vi "configuration UI.vi"() -> ()   [LabVIEW 2014, in "Simple Sequencer TBM editor node.lvclass"]
doc: "This implements the main subpanel functionality for plugging into the Standard Configuration Editor."
uses:
  Simple Sequencer TBM editor node.lvclass
  <vilib>/NI/Configuration Framework/Node/NodeRef.ctl
  <vilib>/NI/Configuration Framework/Node/NISE_CEF_Node.lvclass
  <vilib>/NI/AMC/Message Queue.ctl
  <vilib>/NI/AMC/Message.ctl
  <vilib>/NI/Tools/Keyed Array/KeyedArray.ctl
  <vilib>/NI/Configuration Framework/Node/UserEventRef.ctl
  <vilib>/NI/Configuration Framework/Controls/EventCluster.ctl
  module/configuration/Simple Sequencer TBM configuration.lvclass
  user event typedef.ctl
  VI calling template typedef.ctl
  subpanel state.ctl
  action config and UI pairing.ctl
  sequencer parent classes/action configuration parent/action configuration.lvclass
  module/configuration/Simple Sequencer TBM configuration.lvclass/Simple Sequencer TBM configuration.ctl
  module/configuration/Read sequence definitions.vi
  module/configuration/Read sequencer name.vi
  module/configuration/Write sequencer name.vi
  module/configuration/Read supported actions list VI.vi
  <vilib>/NI/AMC/Create Single Message.vi
  <vilib>/NI/AMC/Update Message Routing Info.vi
  <vilib>/NI/Tag Bus Data Framework/Configuration Editor/Classes/Module editor node/Read Module Configuration.vi
  supported actions list template.vi
  <vilib>/NI/AMC/Send Message.vi
  <vilib>/NI/Tag Bus Module Framework/module configuration/TBM module configuration.lvclass
  <vilib>/NI/Configuration Framework/NISE_CEF_TreeControl.lvlib
  <vilib>/NI/AMC/AMC.lvlib
  <vilib>/NI/Tools/Keyed Array/Tools_KeyedArray.lvlib
panel:
  in  "Settings Button":bool
  in  "Shutdown Action":bool
  in  "Down Button":bool
  in  "Up Button":bool
  in  "Sequencer Name":string
  in  "delete action":bool
  in  "new action":bool
  in  "Actions":i32(listbox)
  in  "delete sequence":bool
  in  "new sequence":bool
  in  "Sequences":i32(listbox)
  in  "user event":T1
  in  "main queue":T2
  in  "node ref":T3
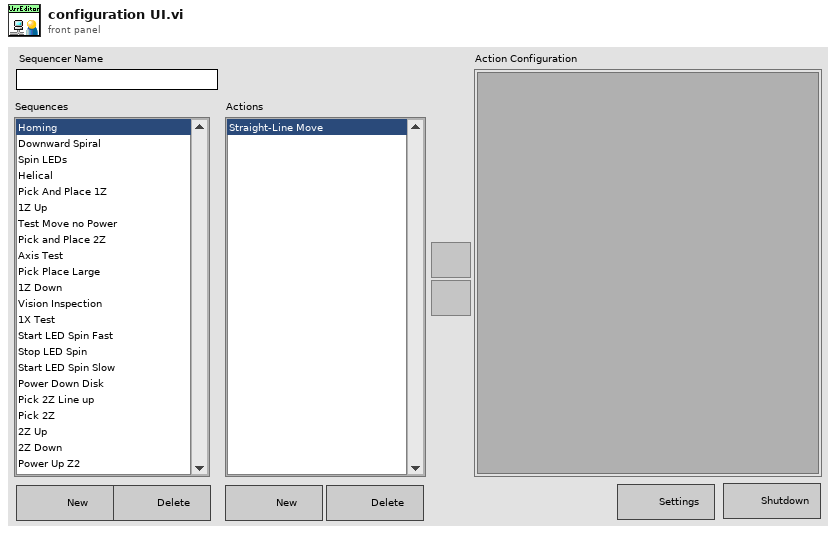
[diagram p1: front panel]
types:
  T1 = typedef "NISE_CEF_Node.lvclass/UserEventRef.ctl" = refnum<user-event>
  T2 = typedef "AMC.lvlib/Message Queue.ctl" = refnum<queue>
  T3 = typedef "NISE_CEF_Node.lvclass/NodeRef.ctl" = refnum<data-value>
  T4 = typedef "Simple Sequencer TBM editor node.lvclass/subpanel state.ctl" = cluster{"active VI":T5, "action UI user event":refnum<user-event>, "SubPnl Refnum":refnum<vi>, "supported actions list":T6[]}
  T5 = typedef "Simple Sequencer TBM editor node.lvclass/VI calling template typedef.ctl" = refnum<vi>
  T6 = typedef "Simple Sequencer TBM editor node.lvclass/action config and UI pairing.ctl" = cluster{"action config":refnum<class "action configuration.lvclass">, "display name":string, "UI VI Path":path}
  T7 = typedef "Simple Sequencer TBM editor node.lvclass/user event typedef.ctl" = cluster{"Message":string, "Data":string}
  T8 = typedef "NISE_CEF_TreeControl.lvlib/EventCluster.ctl" = cluster{"command":string, "data":string}
  T9 = enum8{"Enabled", "Disabled", "Disabled and Grayed Out"}
  T10 = typedef "Simple Sequencer TBM configuration.lvclass/sequence definition.ctl" = cluster{"sequence name":string, "action configs":refnum<class "action configuration.lvclass">[]}
  T11 = typedef "LVPoint32TypeDef.ctl" = cluster{"Horizontal":i32, "Vertical":i32}
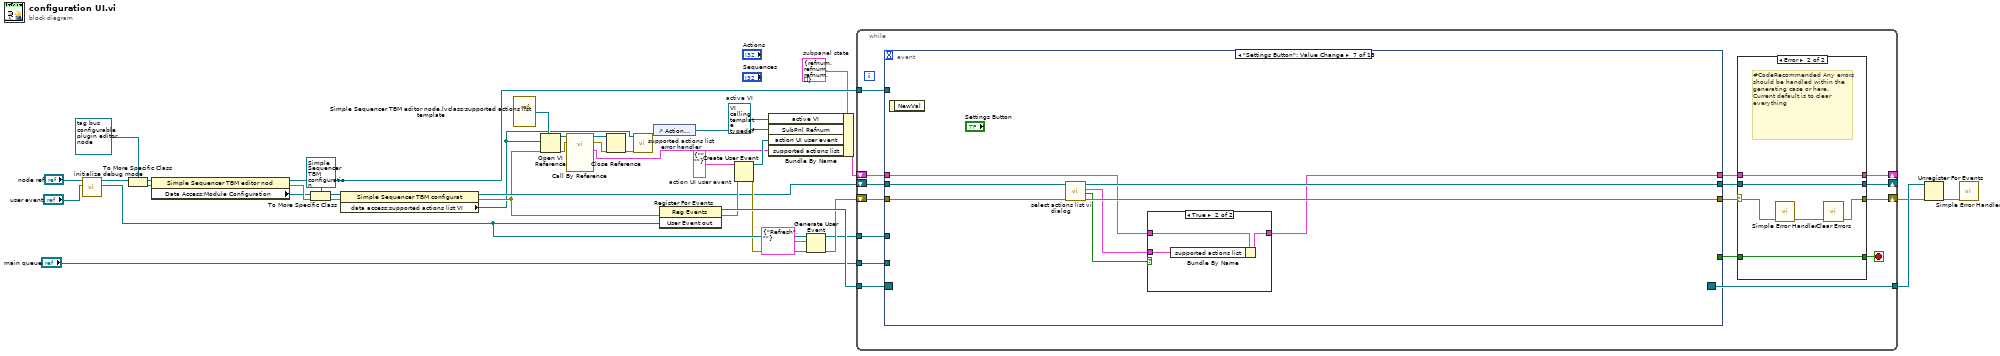
[diagram p0: block diagram]
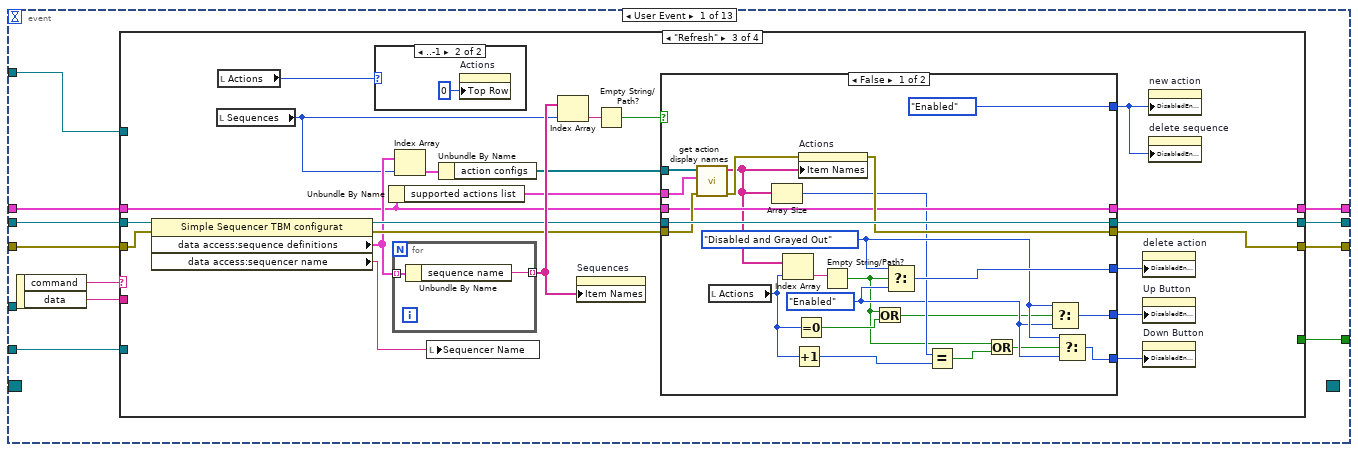
[diagram p3: hidden frame]
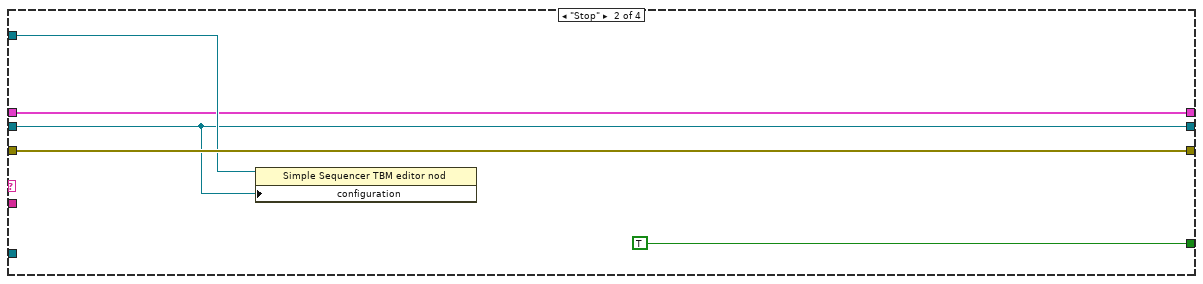
[diagram p5: hidden frame]
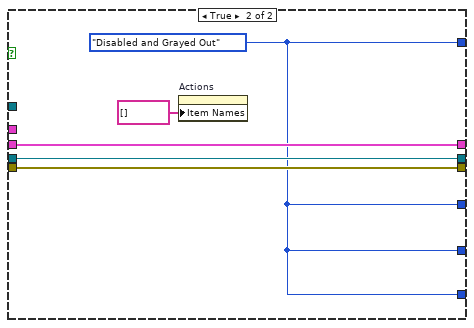
[diagram p7: hidden frame]
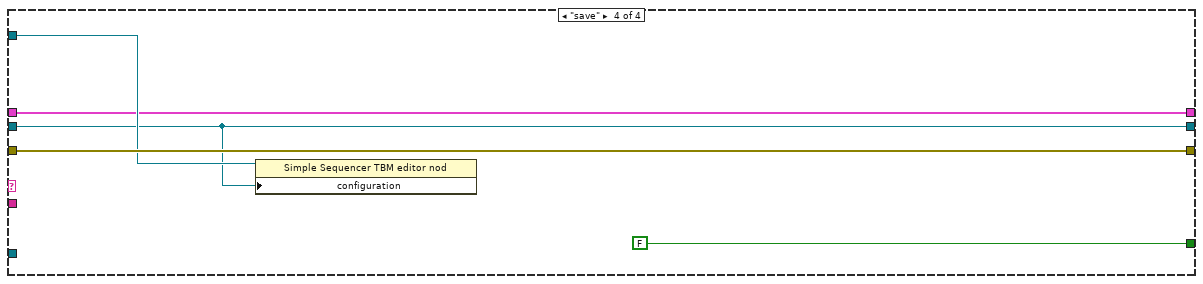
[diagram p8: hidden frame]
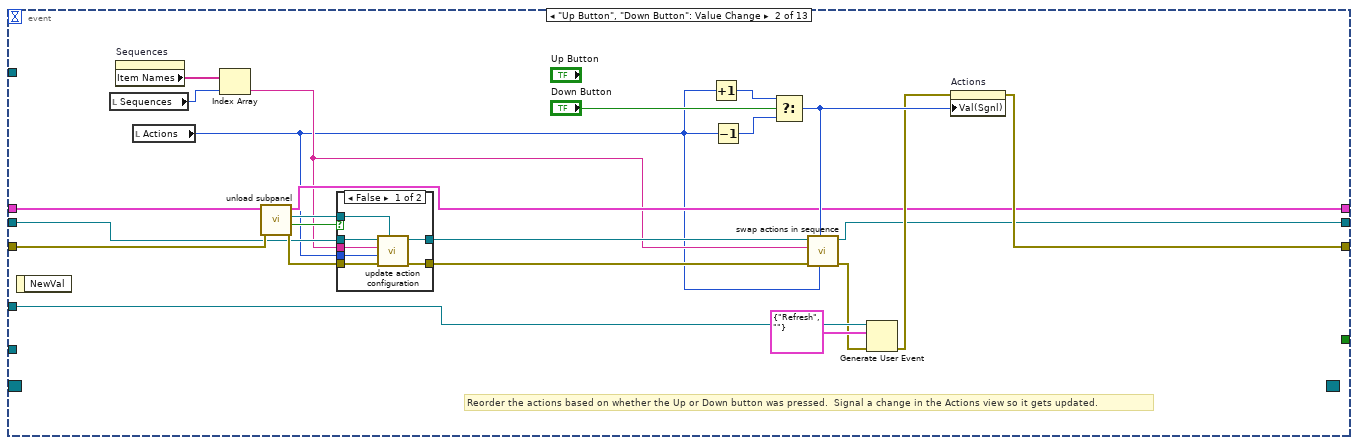
[diagram p9: hidden frame]
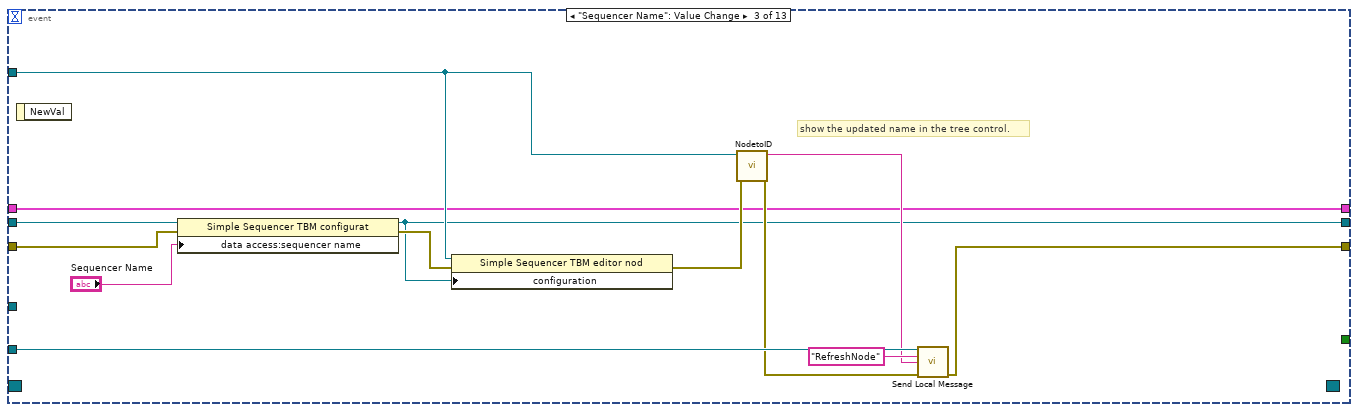
[diagram p11: hidden frame]
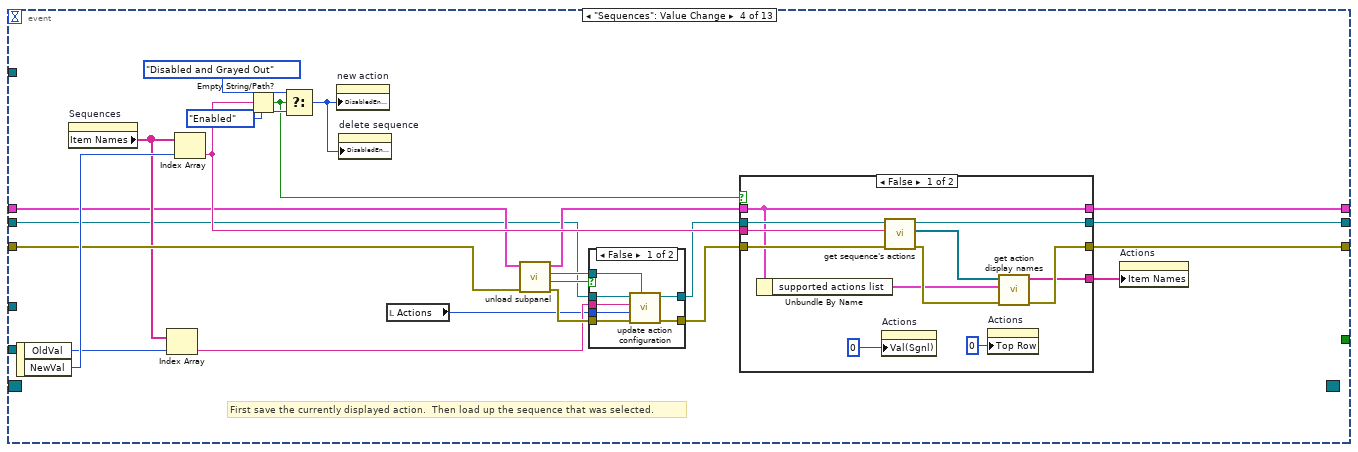
[diagram p12: hidden frame]
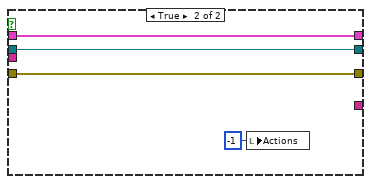
[diagram p14: hidden frame]
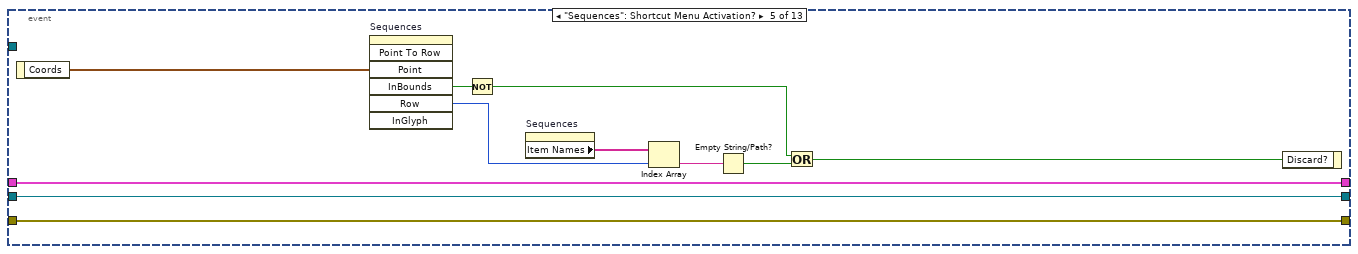
[diagram p15: hidden frame]
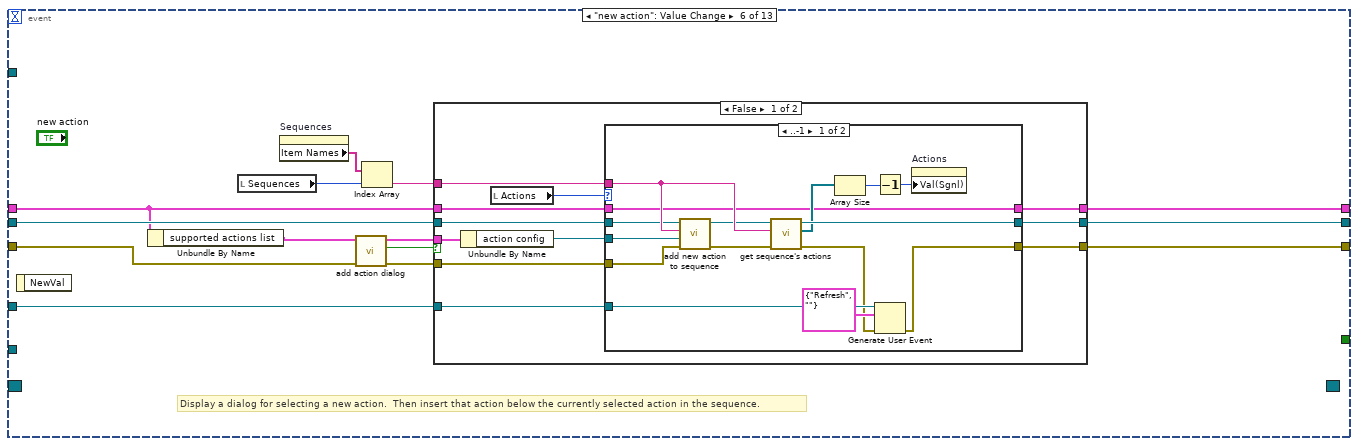
[diagram p16: hidden frame]
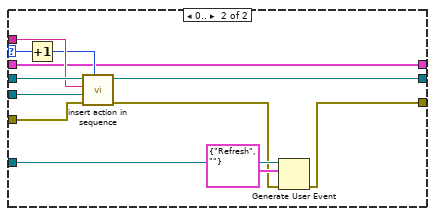
[diagram p17: hidden frame]
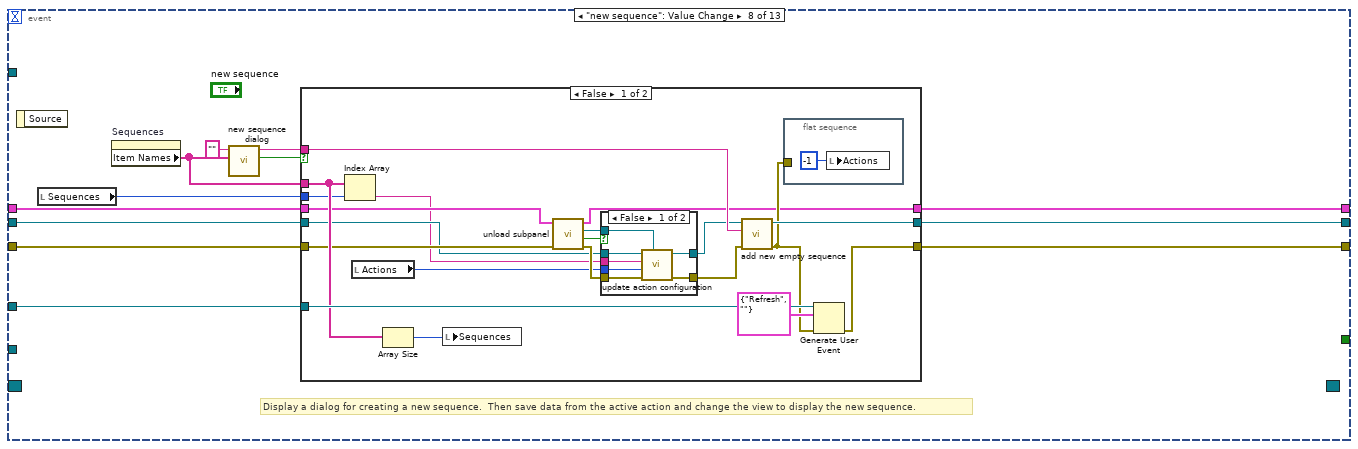
[diagram p20: hidden frame]
diagram:
  w16 = T4 {"active VI"=refnum, "action UI user event"=refnum, "SubPnl Refnum"=refnum, "supported actions list"=[]}  # subpanel state
  w22 = T5 refnum  # active VI
  w23 = T7 {"Message"="", "Data"=""}  # action UI user event
  n1 = call "initialize debug mode.vi"("User Event in"="user event", "editor node in"="node ref") -> ("User Event out"=w27:T1, "editor node out"=w18:T3)  [unwired: 7 in, 1 out]
  n2 = To More Specific Class(target class=refnum<data-value> refnum ("data value reference"), reference=w18) -> (specific class reference=w34:refnum<data-value>, error out=w33:errorcluster)  [unwired: 1 in]
  n3 = property class="Simple Sequencer TBM editor nod"(reference=w34, error in=w33) -> (reference out=w31:refnum<data-value>, error out=w17:errorcluster, "Data Access:Module Configuration"=w10:refnum<class "TBM module configuration.lvclass">)
  n4 = To More Specific Class(target class=refnum<class "Simple Sequencer TBM configuration.lvclass"> refnum ("user module configuration"), reference=w10, error in=w17) -> (specific class reference=w9:refnum<class "Simple Sequencer TBM configuration.lvclass">, error out=w8:errorcluster)
  n5 = property class="Simple Sequencer TBM configurat"(reference=w9, error in=w8) -> (reference out=w7:refnum<class "Simple Sequencer TBM configuration.lvclass">, error out=w6:errorcluster, "data access:supported actions list VI"=w1:path)
  n6 = vi-ref "Simple Sequencer TBM editor node.lvclass:supported actions list template.vi"() -> (w4:refnum<vi>)
  n7 = Open VI Reference(type specifier VI Refnum (for type only)=w4, vi path=w1, error in (no error)=w6) -> (vi reference=w12:refnum<vi>, error out=w3:errorcluster)  [unwired: 3 in]
  n8 = call-by-ref "?"(reference=w12, error in=w3) -> (reference out=w13:refnum<vi>, error out=w11:errorcluster, "supported actions list"=w5:T6[])  [unwired: 11 in]
  n9 = Close Reference(reference=w13, error in (no error)=w11) -> (error out=w2:errorcluster)
  n10 = call "supported actions list error handler.vi"("error in (no error)"=w2, "Path"=w1) -> ()  [unwired: 10 in]
  n11 = control-ref of="Action Configuration"() -> (w14:refnum<vi>)
  n12 = register-events(error in=w6, w27) -> (reference out=w39:refnum<event-registration>, error out=w21:errorcluster)  [unwired: 1 in]
  n13 = Create User Event(user event datatype=w23, error in=w21) -> (user event=w15:refnum<user-event>, error out=w20:errorcluster)
  n14 = Bundle By Name(cluster=w16, "active VI"=w22, "SubPnl Refnum"=w14, "action UI user event"=w15, "supported actions list"=w5) -> (w19:T4)
  n15 = Generate User Event(user event=w27, event data cluster=T8 {"command"="Refresh", "data"=""} ("event data"), error in=w20) -> (user event out=w24:T1, error out=w25:errorcluster)  [unwired: 1 in]
  n16 = while {
    tunnel: w39 -> [w55]
    tunnel: [w54] -> w38
    shift-right: [w50] -> w37
    shift-left: w25 -> [w53]
    shift-right: [w40] -> _
    shift-left: w7 -> [w49]
    tunnel: w31 -> [w47]
    tunnel: "main queue" -> [w46]
    tunnel: w24 -> [w45]
    shift-right: [w42] -> _
    shift-left: w19 -> [w44]
    stop <- w51 stop-if-true
    n17 = event shown="[6] \"Settings Button\": Value Change" {
      selector: w55 -> [_ _ _ _ _ _ _ _ _ _ _ _ _]
      dyn-events: [_ _ _ _ _ _ _ _ _ _ _ _ _] -> w54
      timeout: _ -> [_ _ _ _ _ _ _ _ _ _ _ _ _]
      tunnel: [w74 _ _ _ _ _ _ _ _ _ _ _ _] -> w41
      tunnel: [w75 w155 w184 w204 w246 w254 w306 w321 w363 w446 w499 w533 w572] -> w52
      tunnel: w53 -> [w76 w154 w182 w200 w246 w249 w308 w322 w365 w447 w494 w534 w583]
      tunnel: [w66 w143 w175 w205 w236 w251 w307 w314 w359 w441 w483 w510 w573] -> w48
      tunnel: w49 -> [w72 w149 w187 w192 w236 w250 w309 w323 w366 w448 w488 w517 w578]
      tunnel: w47 -> [w71 _ w177 _ _ _ _ _ _ _ _ _ _]
      tunnel: w46 -> [w70 _ w183 _ _ _ _ _ _ _ _ _ _]
      tunnel: w45 -> [_ w158 _ _ _ w253 _ w319 w362 w444 w498 _ w571]
      tunnel: w44 -> [w68 w153 w176 w197 w237 w248 w304 w318 w361 w443 w493 w521 w582]
      tunnel: [w67 w148 w176 w201 w237 w252 w302 w317 w360 w442 w489 w525 w570] -> w43
      event User Event {
        n18 = event-data() -> ("command"=w73:string, "data"=w69:string)  [unwired: 1 in]
        n19 = case shown="\"Refresh\"" w73 {
          tunnel: [_ TRUE _ FALSE] -> w74
          tunnel: w70 -> [_ _ _ _]
          tunnel: w72 -> [w78 w81 w105 w139]
          tunnel: w76 -> [w79 w83 w106 w141]
          tunnel: [w79 w83 w96 w141] -> w75
          tunnel: w71 -> [_ w82 _ w140]
          tunnel: w69 -> [_ _ _ _]
          tunnel: [w78 w81 w95 w139] -> w66
          tunnel: w68 -> [w77 w80 w86 w138]
          tunnel: [w77 w80 w92 w138] -> w67
          frame Default {
          }
          frame "Stop" {
            n20 = property class="Simple Sequencer TBM editor nod"(reference=w82, "configuration"=w81) -> ()  [unwired: 1 in, 2 out]
          }
          frame "Refresh" {
            n21 = property class="Simple Sequencer TBM configurat"(reference=w105, error in=w106) -> (reference out=w102:refnum<class "Simple Sequencer TBM configuration.lvclass">, error out=w101:errorcluster, "data access:sequence definitions"=w100:T10[], "data access:sequencer name"=w90:string)
            n22 = local read "Sequences"() -> (w99:i32)
            n23 = local read "Actions"() -> (w87:i32)
            n24 = case shown="..-1" w87 {
              frame 0.. {
              }
              frame ..-1 {
                n25 = property on="Actions" class="LstBox (strict)"("Top Row"=0) -> ()  [unwired: 2 in, 2 out]
              }
            }
            n26 = Unbundle By Name(w86) -> ("supported actions list"=w85:T6[])
            n27 = for {
              tunnel: w100 -> [w137] mode=indexing
              tunnel: [w136] -> w104 mode=indexing
              n28 = Unbundle By Name(w137) -> ("sequence name"=w136:string)
            }
            n29 = Index Array(array=w100, index=w99) -> (element=w98:T10)
            n30 = local write "Sequencer Name"(w90) -> ()
            n31 = Unbundle By Name(w98) -> ("action configs"=w97:refnum<class "action configuration.lvclass">[])
            n32 = Index Array(array=w104, index=w99) -> (element=w91:string)
            n33 = property on="Sequences" class="LstBox (strict)"("Item Names"=w104) -> ()  [unwired: 2 in, 2 out]
            n34 = Empty String/Path?(string/path=w91) -> (empty?=w103:bool)
            n35 = case shown="False" w103 {
              tunnel: [T9."Enabled" ("Disabled") w131] -> w94
              tunnel: w102 -> [w129 w135]
              tunnel: w101 -> [w126 w134]
              tunnel: w97 -> [w127 _]
              tunnel: [w125 w134] -> w96
              tunnel: [w129 w135] -> w95
              tunnel: [w123 w131] -> w93
              tunnel: w86 -> [w122 w132]
              tunnel: [w122 w132] -> w92
              tunnel: [w120 w131] -> w89
              tunnel: [w115 w131] -> w88
              tunnel: w85 -> [w108 _]
              frame False {
                w119 = T9."Disabled and Grayed Out" ("t")
                w114 = T9."Enabled" ("Disabled")
                n36 = call "get action display names.vi"("error in (no error)"=w126, "supported actions list"=w108, "action configs"=w127) -> ("error out"=w128:errorcluster, "display names"=w117:string[])  [unwired: 7 in]
                n37 = local read "Actions"() -> (w121:i32)
                n38 = Array Size(array=w117) -> (size(s)=w116:i32)
                n39 = Index Array(array=w117, index=w121) -> (element=w124:string)
                n40 = Increment(x=w121) -> (x+1=w118:i32)
                n41 = Equal To 0?(x=w121) -> (x = 0?=w113:bool)
                n42 = property on="Actions" class="LstBox (strict)"(error in=w128, "Item Names"=w117) -> (error out=w125:errorcluster)  [unwired: 1 in, 1 out]
                n43 = Empty String/Path?(string/path=w124) -> (empty?=w110:bool)
                n44 = Or(x=w110, y=w113) -> (x .or. y?=w112:bool)
                n45 = Select(t=w119, s=w110, f=w114) -> (s? t:f=w123:T9)
                n46 = Equal?(x=w116, y=w118) -> (x = y?=w111:bool)
                n47 = Or(x=w110, y=w111) -> (x .or. y?=w109:bool)
                n48 = Select(t=w119, s=w112, f=w114) -> (s? t:f=w120:T9)
                n49 = Select(t=w119, s=w109, f=w114) -> (s? t:f=w115:T9)
              }
              frame True {
                w131 = T9."Disabled and Grayed Out" ("Disabled")
                n50 = property on="Actions" class="LstBox (strict)"("Item Names"=string[] []) -> ()  [unwired: 2 in, 2 out]
              }
            }
            n51 = property on="delete action" class="Bool"("DisabledEnum"=w93) -> ()  [unwired: 2 in, 2 out]
            n52 = property on="Up Button" class="Bool"("DisabledEnum"=w89) -> ()  [unwired: 2 in, 2 out]
            n53 = property on="Down Button" class="Bool"("DisabledEnum"=w88) -> ()  [unwired: 2 in, 2 out]
            n54 = property on="new action" class="Bool"("DisabledEnum"=w94) -> ()  [unwired: 2 in, 2 out]
            n55 = property on="delete sequence" class="Bool"("DisabledEnum"=w94) -> ()  [unwired: 2 in, 2 out]
          }
          frame "save" {
            n56 = property class="Simple Sequencer TBM editor nod"(reference=w140, "configuration"=w139) -> ()  [unwired: 1 in, 2 out]
          }
        }
      }
      event "Up Button", "Down Button": Value Change {
        # "Reorder the actions based on whether the Up or Down button was pressed.  Signal a change in the Actions view so it gets updated."
        n57 = event-data() -> ()  [unwired: 1 in, 1 out]
        n58 = local read "Sequences"() -> (w161:i32)
        n59 = property on="Sequences" class="LstBox (strict)"() -> ("Item Names"=w162:string[])  [unwired: 2 in, 2 out]
        n60 = local read "Actions"() -> (w144:i32)
        n61 = Index Array(array=w162, index=w161) -> (element=w146:string)
        n62 = call "unload subpanel.vi"("error in (no error)"=w154, "subpanel state"=w153) -> ("error out"=w150:errorcluster, "empty?"=w151:bool, "action configuration out"=w152:refnum<class "action configuration.lvclass">, "subpanel state out"=w148:T4)  [unwired: 6 in]
        n63 = case shown="False" w151 {
          tunnel: w152 -> [w172 _]
          tunnel: w149 -> [w171 w174]
          tunnel: w144 -> [w170 _]
          tunnel: w146 -> [w169 _]
          tunnel: w150 -> [w168 w173]
          tunnel: [w167 w174] -> w147
          tunnel: [w166 w173] -> w145
          frame False {
            n64 = call "update action configuration.vi"("action config"=w172, "error in (no error)"=w168, "index"=w170, "sequence name"=w169, "Simple Sequencer TBM configuration in"=w171) -> ("error out"=w166:errorcluster, "Simple Sequencer TBM configuration out"=w167:refnum<class "Simple Sequencer TBM configuration.lvclass">)  [unwired: 5 in]
          }
          frame True {
          }
        }
        n65 = Increment(x=w144) -> (x+1=w165:i32)
        n66 = Decrement(x=w144) -> (x-1=w164:i32)
        n67 = Select(t=w165, s="Down Button", f=w164) -> (s? t:f=w160:i32)
        n68 = call "swap actions in sequence.vi"("action index 2"=w144, "action index 1"=w160, "error in (no error)"=w145, "sequence name"=w146, "Simple Sequencer TBM configuration in"=w147) -> ("error out"=w157:errorcluster, "Simple Sequencer TBM configuration out"=w143:refnum<class "Simple Sequencer TBM configuration.lvclass">)  [unwired: 5 in]
        n69 = Generate User Event(user event=w158, event data cluster=T8 {"command"="Refresh", "data"=""} ("event data"), error in=w157) -> (error out=w156:errorcluster)  [unwired: 1 in, 1 out]
        n70 = property on="Actions" class="LstBox (strict)"(error in=w156, "Val(Sgnl)"=w160) -> (error out=w155:errorcluster)  [unwired: 1 in, 1 out]
      }
      event "Sequencer Name": Value Change {
        # "show the updated name in the tree control."
        n71 = event-data() -> ()  [unwired: 1 in, 1 out]
        n72 = property class="Simple Sequencer TBM configurat"(reference=w187, error in=w182, "data access:sequencer name"="Sequencer Name") -> (reference out=w175:refnum<class "Simple Sequencer TBM configuration.lvclass">, error out=w179:errorcluster)
        n73 = property class="Simple Sequencer TBM editor nod"(reference=w177, error in=w179, "configuration"=w175) -> (error out=w178:errorcluster)  [unwired: 1 out]
        n74 = call <vilib>:"NodetoID.vi"("error in"=w178, "node ref"=w177) -> ("error out"=w181:errorcluster, "ID"=w180:string)  [unwired: 8 in]
        n75 = call <vilib>:"Send Local Message.vi"("message queue in"=w183, "message name"="RefreshNode", "message value"=w180, "error in"=w181) -> ("error out"=w184:errorcluster)  [unwired: 9 in, 2 out]
      }
      event "Sequences": Value Change {
        # "First save the currently displayed action.  Then load up the sequence that was selected."
        n76 = event-data() -> ("OldVal"=w198:i32, "NewVal"=w210:i32)  [unwired: 1 in]
        n77 = property on="Sequences" class="LstBox (strict)"() -> ("Item Names"=w199:string[])  [unwired: 2 in, 2 out]
        n78 = Index Array(array=w199, index=w198) -> (element=w189:string)
        n79 = Index Array(array=w199, index=w210) -> (element=w206:string)
        n80 = Empty String/Path?(string/path=w206) -> (empty?=w207:bool)
        n81 = Select(t=T9."Disabled and Grayed Out" ("Disabled"), s=w207, f=T9."Enabled" ("Disabled")) -> (s? t:f=w203:T9)
        n82 = property on="new action" class="Bool"("DisabledEnum"=w203) -> ()  [unwired: 2 in, 2 out]
        n83 = property on="delete sequence" class="Bool"("DisabledEnum"=w203) -> ()  [unwired: 2 in, 2 out]
        n84 = local read "Actions"() -> (w188:i32)
        n85 = call "unload subpanel.vi"("error in (no error)"=w200, "subpanel state"=w197) -> ("error out"=w193:errorcluster, "empty?"=w195:bool, "action configuration out"=w194:refnum<class "action configuration.lvclass">, "subpanel state out"=w196:T4)  [unwired: 6 in]
        n86 = case shown="False" w195 {
          tunnel: w194 -> [w217 _]
          tunnel: w192 -> [w216 w219]
          tunnel: w188 -> [w215 _]
          tunnel: w189 -> [w214 _]
          tunnel: w193 -> [w213 w218]
          tunnel: [w212 w219] -> w191
          tunnel: [w211 w218] -> w190
          frame False {
            n87 = call "update action configuration.vi"("action config"=w217, "error in (no error)"=w213, "index"=w215, "sequence name"=w214, "Simple Sequencer TBM configuration in"=w216) -> ("error out"=w211:errorcluster, "Simple Sequencer TBM configuration out"=w212:refnum<class "Simple Sequencer TBM configuration.lvclass">)  [unwired: 5 in]
          }
          frame True {
          }
        }
        n88 = case shown="False" w207 {
          tunnel: w191 -> [w223 w235]
          tunnel: w206 -> [w231 _]
          tunnel: w190 -> [w230 w234]
          tunnel: [w222 w235] -> w205
          tunnel: [w227 w234] -> w204
          tunnel: [w226 _] -> w202
          tunnel: w196 -> [w221 w233]
          tunnel: [w221 w233] -> w201
          frame False {
            n89 = Unbundle By Name(w221) -> ("supported actions list"=w220:T6[])
            n90 = property on="Actions" class="LstBox (strict)"("Val(Sgnl)"=0 ("Actions")) -> ()  [unwired: 2 in, 2 out]
            n91 = call "get sequence's actions.vi"("error in (no error)"=w230, "sequence name"=w231, "Simple Sequencer TBM configuration in"=w223) -> ("error out"=w228:errorcluster, "action configs"=w229:refnum<class "action configuration.lvclass">[], "Simple Sequencer TBM configuration out"=w222:refnum<class "Simple Sequencer TBM configuration.lvclass">)  [unwired: 6 in]
            n92 = property on="Actions" class="LstBox (strict)"("Top Row"=0) -> ()  [unwired: 2 in, 2 out]
            n93 = call "get action display names.vi"("error in (no error)"=w228, "supported actions list"=w220, "action configs"=w229) -> ("error out"=w227:errorcluster, "display names"=w226:string[])  [unwired: 7 in]
          }
          frame True {
            n94 = local write "Actions"(-1 ("Actions")) -> ()
          }
        }
        n95 = property on="Actions" class="LstBox (strict)"("Item Names"=w202) -> ()  [unwired: 2 in, 2 out]
      }
      event "Sequences": Shortcut Menu Activation? {
        n96 = event-data() -> ("Coords"=w243:T11)  [unwired: 1 in]
        n97 = invoke on="Sequences" class="LstBox (strict)" method="Point To Row"("Point"=w243) -> ("InBounds"=w241:bool, "Row"=w242:i32)  [unwired: 6 in, 5 out]
        n98 = Not(x=w241) -> (.not. x?=w239:bool)
        n99 = property on="Sequences" class="LstBox (strict)"() -> ("Item Names"=w245:string[])  [unwired: 2 in, 2 out]
        n100 = Index Array(array=w245, index=w242) -> (element=w244:string)
        n101 = Empty String/Path?(string/path=w244) -> (empty?=w240:bool)
        n102 = Or(x=w239, y=w240) -> (x .or. y?=w238:bool)
        n103 = event-data("Discard?"=w238) -> ()  [unwired: 1 in, 1 out]
      }
      event "new action": Value Change {
        # "Display a dialog for selecting a new action.  Then insert that action below the currently selected action in the sequence."
        n104 = event-data() -> ()  [unwired: 1 in, 1 out]
        n105 = Unbundle By Name(w248) -> ("supported actions list"=w247:T6[])
        n106 = local read "Sequences"() -> (w256:i32)
        n107 = property on="Sequences" class="LstBox (strict)"() -> ("Item Names"=w257:string[])  [unwired: 2 in, 2 out]
        n108 = call "add action dialog.vi"("error in (no error)"=w249, "supported actions list"=w247) -> ("error out"=w260:errorcluster, "cancelled"=w259:bool, "config and UI pairing"=w258:T6)  [unwired: 7 in]
        n109 = Index Array(array=w257, index=w256) -> (element=w255:string)
        n110 = case shown="False" w259 {
          tunnel: w260 -> [w266 w300]
          tunnel: [w268 w301] -> w251
          tunnel: w250 -> [w267 w301]
          tunnel: w258 -> [w271 _]
          tunnel: w255 -> [w263 _]
          tunnel: [w269 w300] -> w254
          tunnel: w253 -> [w270 _]
          tunnel: w248 -> [w262 w299]
          tunnel: [w261 w299] -> w252
          frame False {
            n111 = Unbundle By Name(w271) -> ("action config"=w265:refnum<class "action configuration.lvclass">)
            n112 = local read "Actions"() -> (w264:i32)
            n113 = case shown="..-1" w264 {
              selector: w264 -> [_ w292]
              tunnel: w270 -> [w285 w297]
              tunnel: [w284 w296] -> w269
              tunnel: [w282 w289] -> w268
              tunnel: w267 -> [w274 w295]
              tunnel: w266 -> [w277 w294]
              tunnel: w265 -> [w276 w293]
              tunnel: w263 -> [w275 w291]
              tunnel: w262 -> [w272 w287]
              tunnel: [w272 w287] -> w261
              frame ..-1 {
                n114 = call "add new action to sequence.vi"("error in (no error)"=w277, "new action"=w276, "sequence name"=w275, "Simple Sequencer TBM configuration in"=w274) -> ("error out"=w278:errorcluster, "Simple Sequencer TBM configuration out"=w273:refnum<class "Simple Sequencer TBM configuration.lvclass">)  [unwired: 6 in]
                n115 = call "get sequence's actions.vi"("error in (no error)"=w278, "sequence name"=w275, "Simple Sequencer TBM configuration in"=w273) -> ("error out"=w283:errorcluster, "action configs"=w280:refnum<class "action configuration.lvclass">[], "Simple Sequencer TBM configuration out"=w282:refnum<class "Simple Sequencer TBM configuration.lvclass">)  [unwired: 6 in]
                n116 = Array Size(array=w280) -> (size(s)=w281:i32)
                n117 = Decrement(x=w281) -> (x-1=w279:i32)
                n118 = Generate User Event(user event=w285, event data cluster=T8 {"command"="Refresh", "data"=""} ("event data"), error in=w283) -> (error out=w284:errorcluster)  [unwired: 1 in, 1 out]
                n119 = property on="Actions" class="LstBox (strict)"("Val(Sgnl)"=w279) -> ()  [unwired: 2 in, 2 out]
              }
              frame 0.. {
                n120 = Increment(x=w292) -> (x+1=w290:i32)
                n121 = call "insert action in sequence.vi"("index"=w290, "error in (no error)"=w294, "new action"=w293, "sequence name"=w291, "Simple Sequencer TBM configuration in"=w295) -> ("error out"=w288:errorcluster, "Simple Sequencer TBM configuration out"=w289:refnum<class "Simple Sequencer TBM configuration.lvclass">)  [unwired: 5 in]
                n122 = Generate User Event(user event=w297, event data cluster=T8 {"command"="Refresh", "data"=""} ("event data"), error in=w288) -> (error out=w296:errorcluster)  [unwired: 1 in, 1 out]
              }
            }
          }
          frame True {
          }
        }
      }
      event "Settings Button": Value Change {
        n123 = event-data() -> ()  [unwired: 1 in, 1 out]
        n124 = call "select actions list vi dialog.vi"("error in (no error)"=w308, "sequencer configuration"=w309) -> ("error out"=w306:errorcluster, "success?"=w305:bool, "supported actions list"=w303:T6[], "sequencer configuration out"=w307:refnum<class "Simple Sequencer TBM configuration.lvclass">)  [unwired: 6 in]
        n125 = case shown="True" w305 {
          tunnel: w304 -> [w310 w313]
          tunnel: w303 -> [_ w312]
          tunnel: [w310 w311] -> w302
          frame False {
          }
          frame True {
            n126 = Bundle By Name(cluster=w313, "supported actions list"=w312) -> (w311:T4)
          }
        }
      }
      event "new sequence": Value Change {
        # "Display a dialog for creating a new sequence.  Then save data from the active action and change the view to display the new sequence."
        n127 = event-data() -> ()  [unwired: 1 in, 1 out]
        n128 = local read "Sequences"() -> (w315:i32)
        n129 = property on="Sequences" class="LstBox (strict)"() -> ("Item Names"=w316:string[])  [unwired: 2 in, 2 out]
        n130 = call "new sequence dialog.vi"("Existing Sequences"=w316, "Sequence Name"="") -> ("Canceled?"=w324:bool, "Sequence Name Out"=w320:string)  [unwired: 8 in]
        n131 = case shown="False" w324 {
          tunnel: w323 -> [w330 w358]
          tunnel: w322 -> [w338 w357]
          tunnel: [w341 w358] -> w314
          tunnel: [w344 w357] -> w321
          tunnel: w320 -> [w342 _]
          tunnel: w319 -> [w343 _]
          tunnel: w318 -> [w335 w356]
          tunnel: [w334 w356] -> w317
          tunnel: w316 -> [w340 _]
          tunnel: w315 -> [w339 _]
          frame False {
            n132 = Index Array(array=w340, index=w339) -> (element=w329:string)
            n133 = local read "Actions"() -> (w328:i32)
            n134 = Array Size(array=w340) -> (size(s)=w337:i32)
            n135 = local write "Sequences"(w337) -> ()
            n136 = call "unload subpanel.vi"("error in (no error)"=w338, "subpanel state"=w335) -> ("error out"=w331:errorcluster, "empty?"=w332:bool, "action configuration out"=w333:refnum<class "action configuration.lvclass">, "subpanel state out"=w334:T4)  [unwired: 6 in]
            n137 = case shown="False" w332 {
              tunnel: w333 -> [w352 _]
              tunnel: w330 -> [w351 w354]
              tunnel: w328 -> [w350 _]
              tunnel: w329 -> [w349 _]
              tunnel: w331 -> [w348 w353]
              tunnel: [w347 w354] -> w327
              tunnel: [w346 w353] -> w326
              frame False {
                n138 = call "update action configuration.vi"("action config"=w352, "error in (no error)"=w348, "index"=w350, "sequence name"=w349, "Simple Sequencer TBM configuration in"=w351) -> ("error out"=w346:errorcluster, "Simple Sequencer TBM configuration out"=w347:refnum<class "Simple Sequencer TBM configuration.lvclass">)  [unwired: 5 in]
              }
              frame True {
              }
            }
            n139 = call "add new empty sequence.vi"("error in (no error)"=w326, "sequence name"=w342, "Simple Sequencer TBM configuration in"=w327) -> ("error out"=w336:errorcluster, "Simple Sequencer TBM configuration out"=w341:refnum<class "Simple Sequencer TBM configuration.lvclass">)  [unwired: 7 in]
            n140 = flat-sequence {
              tunnel: w336 -> [_]
              frame #0 {
                n141 = local write "Actions"(-1 ("Actions")) -> ()
              }
            }
            n142 = Generate User Event(user event=w343, event data cluster=T8 {"command"="Refresh", "data"=""} ("event data"), error in=w336) -> (error out=w344:errorcluster)  [unwired: 1 in, 1 out]
          }
          frame True {
          }
        }
      }
      event "Sequences": Shortcut Menu Selection (User) {
        n143 = event-data() -> ("ItemTag"=w367:string, "Coords"=w364:T11)  [unwired: 1 in]
        n144 = case shown="Default" w367 {
          tunnel: w366 -> [w370 w379 w403]
          tunnel: w365 -> [w369 w378 w424]
          tunnel: w364 -> [_ w383 w425]
          tunnel: [w370 w376 w416] -> w359
          tunnel: [w369 w375 w414] -> w363
          tunnel: w362 -> [_ w374 _]
          tunnel: w361 -> [w368 w372 w407]
          tunnel: [w368 w371 w398] -> w360
          frame Default {
          }
          frame "Edit".. {
            n145 = invoke on="Sequences" class="LstBox (strict)" method="Point To Row"("Point"=w383) -> ("Row"=w384:i32)  [unwired: 6 in, 6 out]
            n146 = property on="Sequences" class="LstBox (strict)"(error in=w378) -> (error out=w377:errorcluster, "Item Names"=w382:string[])  [unwired: 1 in, 1 out]
            n147 = Index Array(array=w382, index=w384) -> (element=w373:string)
            n148 = call "new sequence dialog.vi"("Existing Sequences"=w382, "Sequence Name"=w373) -> ("Canceled?"=w381:bool, "Sequence Name Out"=w380:string)  [unwired: 8 in]
            n149 = case shown="False" w381 {
              tunnel: w380 -> [w386 _]
              tunnel: w379 -> [w391 w397]
              tunnel: w377 -> [w389 w396]
              tunnel: [w390 w397] -> w376
              tunnel: [w393 w396] -> w375
              tunnel: w374 -> [w392 _]
              tunnel: w373 -> [w387 _]
              tunnel: w372 -> [w385 w395]
              tunnel: [w385 w395] -> w371
              frame False {
                n150 = call "rename sequence.vi"("error in (no error)"=w389, "new sequence name"=w386, "old sequence name"=w387, "Simple Sequencer TBM configuration in"=w391) -> ("error out"=w388:errorcluster, "Simple Sequencer TBM configuration out"=w390:refnum<class "Simple Sequencer TBM configuration.lvclass">)  [unwired: 6 in]
                n151 = Generate User Event(user event=w392, event data cluster=T8 {"command"="Refresh", "data"=""} ("event data"), error in=w388) -> (error out=w393:errorcluster)  [unwired: 1 in, 1 out]
              }
              frame True {
              }
            }
          }
          frame "Duplicate.." {
            n152 = invoke on="Sequences" class="LstBox (strict)" method="Point To Row"(error in=w424, "Point"=w425) -> (error out=w408:errorcluster, "Row"=w423:i32)  [unwired: 5 in, 5 out]
            n153 = property on="Sequences" class="LstBox (strict)"() -> ("Item Names"=w411:string[])  [unwired: 2 in, 2 out]
            n154 = local read "Actions"() -> (w402:i32)
            n155 = Index Array(array=w411, index=w423) -> (element=w399:string)
            n156 = call "unload subpanel.vi"("error in (no error)"=w408, "subpanel state"=w407) -> ("error out"=w404:errorcluster, "empty?"=w406:bool, "action configuration out"=w405:refnum<class "action configuration.lvclass">, "subpanel state out"=w398:T4)  [unwired: 6 in]
            n157 = case shown="False" w406 {
              tunnel: w405 -> [w432 _]
              tunnel: w403 -> [w431 w434]
              tunnel: w402 -> [w430 _]
              tunnel: w399 -> [w429 _]
              tunnel: w404 -> [w428 w433]
              tunnel: [w427 w434] -> w401
              tunnel: [w426 w433] -> w400
              frame False {
                n158 = call "update action configuration.vi"("action config"=w432, "error in (no error)"=w428, "index"=w430, "sequence name"=w429, "Simple Sequencer TBM configuration in"=w431) -> ("error out"=w426:errorcluster, "Simple Sequencer TBM configuration out"=w427:refnum<class "Simple Sequencer TBM configuration.lvclass">)  [unwired: 5 in]
              }
              frame True {
              }
            }
            n159 = Concatenate Strings(w399, " Dup" ("string")) -> (w410:string)
            n160 = call "get sequence's actions.vi"("error in (no error)"=w400, "sequence name"=w399, "Simple Sequencer TBM configuration in"=w401) -> ("error out"=w420:errorcluster, "action configs"=w417:refnum<class "action configuration.lvclass">[], "Simple Sequencer TBM configuration out"=w421:refnum<class "Simple Sequencer TBM configuration.lvclass">)  [unwired: 6 in]
            n161 = Build Array (concatenate)(w411, w410) -> (w409:string[])
            n162 = Array Size(array=w411) -> (size(s)=w415:i32)
            n163 = call "add new empty sequence.vi"("error in (no error)"=w420, "sequence name"=w410, "Simple Sequencer TBM configuration in"=w421) -> ("error out"=w418:errorcluster, "Simple Sequencer TBM configuration out"=w419:refnum<class "Simple Sequencer TBM configuration.lvclass">)  [unwired: 7 in]
            n164 = for {
              shift-right: [w439] -> w416
              shift-left: w419 -> [w440]
              shift-right: [w437] -> w413
              shift-left: w418 -> [w438]
              tunnel: w410 -> [w436]
              tunnel: w417 -> [w435] mode=indexing
              n165 = call "add new action to sequence.vi"("error in (no error)"=w438, "new action"=w435, "sequence name"=w436, "Simple Sequencer TBM configuration in"=w440) -> ("error out"=w437:errorcluster, "Simple Sequencer TBM configuration out"=w439:refnum<class "Simple Sequencer TBM configuration.lvclass">)  [unwired: 6 in]
            }
            n166 = property on="Sequences" class="LstBox (strict)"(error in=w413, "Item Names"=w409) -> (error out=w412:errorcluster)  [unwired: 1 in, 1 out]
            n167 = property on="Sequences" class="LstBox (strict)"(error in=w412, "Val(Sgnl)"=w415) -> (error out=w414:errorcluster)  [unwired: 1 in, 1 out]
          }
        }
      }
      event "delete sequence": Value Change {
        # "Verify that this was done intentionally.  Then save the currently selected action and delete the sequence if approved."
        n168 = event-data() -> ()  [unwired: 1 in, 1 out]
        n169 = property on="Sequences" class="LstBox (strict)"() -> ("Item Names"=w454:string[])  [unwired: 2 in, 2 out]
        n170 = local read "Sequences"() -> (w453:i32)
        n171 = Index Array(array=w454, index=w453) -> (element=w445:string)
        n172 = Concatenate Strings("Are you sure you would like to delete '", w445, "'?" ("string")) -> (w450:string)
        n173 = Two Button Dialog(message=w450) -> (T button?=w449:bool)  [unwired: 2 in]
        n174 = case shown="False" w449 {
          tunnel: w448 -> [w457 w462]
          tunnel: [w457 w473] -> w441
          tunnel: w447 -> [w456 w469]
          tunnel: [w456 w470] -> w446
          tunnel: w445 -> [_ w459]
          tunnel: w444 -> [_ w468]
          tunnel: w443 -> [w455 w467]
          tunnel: [w455 w458] -> w442
          frame False {
          }
          frame True {
            n175 = local read "Actions"() -> (w463:i32)
            n176 = call "unload subpanel.vi"("error in (no error)"=w469, "subpanel state"=w467) -> ("error out"=w464:errorcluster, "empty?"=w465:bool, "action configuration out"=w466:refnum<class "action configuration.lvclass">, "subpanel state out"=w458:T4)  [unwired: 6 in]
            n177 = case shown="False" w465 {
              tunnel: w466 -> [w480 _]
              tunnel: w462 -> [w479 w482]
              tunnel: w463 -> [w478 _]
              tunnel: w459 -> [w477 _]
              tunnel: w464 -> [w476 w481]
              tunnel: [w475 w482] -> w461
              tunnel: [w474 w481] -> w460
              frame False {
                n178 = call "update action configuration.vi"("action config"=w480, "error in (no error)"=w476, "index"=w478, "sequence name"=w477, "Simple Sequencer TBM configuration in"=w479) -> ("error out"=w474:errorcluster, "Simple Sequencer TBM configuration out"=w475:refnum<class "Simple Sequencer TBM configuration.lvclass">)  [unwired: 5 in]
              }
              frame True {
              }
            }
            n179 = call "delete sequence.vi"("error in (no error)"=w460, "sequence name"=w459, "Simple Sequencer TBM configuration in"=w461) -> ("error out"=w471:errorcluster, "Simple Sequencer TBM configuration out"=w473:refnum<class "Simple Sequencer TBM configuration.lvclass">)  [unwired: 7 in]
            n180 = Generate User Event(user event=w468, event data cluster=T8 {"command"="Refresh", "data"=""} ("event data"), error in=w471) -> (error out=w470:errorcluster)  [unwired: 1 in, 1 out]
          }
        }
      }
      event "delete action": Value Change {
        n181 = event-data() -> ()  [unwired: 1 in, 2 out]
        n182 = local read "Sequences"() -> (w500:i32)
        n183 = property on="Sequences" class="LstBox (strict)"() -> ("Item Names"=w496:string[])  [unwired: 2 in, 2 out]
        n184 = Index Array(array=w496, index=w500) -> (element=w485:string)
        n185 = local read "Actions"() -> (w484:i32)
        n186 = call "unload subpanel.vi"("error in (no error)"=w494, "subpanel state"=w493) -> ("error out"=w490:errorcluster, "empty?"=w491:bool, "action configuration out"=w492:refnum<class "action configuration.lvclass">, "subpanel state out"=w489:T4)  [unwired: 6 in]
        n187 = case shown="False" w491 {
          tunnel: w492 -> [w507 _]
          tunnel: w488 -> [w506 w509]
          tunnel: w484 -> [w505 _]
          tunnel: w485 -> [w504 _]
          tunnel: w490 -> [w503 w508]
          tunnel: [w502 w509] -> w487
          tunnel: [w501 w508] -> w486
          frame False {
            n188 = call "update action configuration.vi"("action config"=w507, "error in (no error)"=w503, "index"=w505, "sequence name"=w504, "Simple Sequencer TBM configuration in"=w506) -> ("error out"=w501:errorcluster, "Simple Sequencer TBM configuration out"=w502:refnum<class "Simple Sequencer TBM configuration.lvclass">)  [unwired: 5 in]
          }
          frame True {
          }
        }
        n189 = call "delete action from sequence by index.vi"("error in (no error)"=w486, "index"=w484, "sequence name"=w485, "Simple Sequencer TBM configuration in"=w487) -> ("error out"=w495:errorcluster, "Simple Sequencer TBM configuration out"=w483:refnum<class "Simple Sequencer TBM configuration.lvclass">)  [unwired: 6 in]
        n190 = Generate User Event(user event=w498, event data cluster=T8 {"command"="Refresh", "data"=""} ("event data"), error in=w495) -> (error out=w499:errorcluster)  [unwired: 1 in, 1 out]
      }
      event "Actions": Value Change {
        # "Redraw the actions view based on data in the configuration class.  First save the data associated with the currently selected action. Then load up the newly selected one."
        n191 = event-data() -> ("NewVal"=w516:i32, "OldVal"=w515:i32)  [unwired: 1 in]
        n192 = local read "Sequences"() -> (w532:i32)
        n193 = property on="Sequences" class="LstBox (strict)"() -> ("Item Names"=w531:string[])  [unwired: 2 in, 2 out]
        n194 = call "unload subpanel.vi"("error in (no error)"=w534, "subpanel state"=w521) -> ("error out"=w514:errorcluster, "empty?"=w519:bool, "action configuration out"=w518:refnum<class "action configuration.lvclass">, "subpanel state out"=w520:T4)  [unwired: 6 in]
        n195 = Index Array(array=w531, index=w532) -> (element=w511:string)
        n196 = case shown="True" w519 {
          tunnel: w518 -> [w541 _]
          tunnel: w517 -> [w540 w543]
          tunnel: w515 -> [w539 _]
          tunnel: w511 -> [w538 _]
          tunnel: w514 -> [w537 w542]
          tunnel: [w536 w543] -> w513
          tunnel: [w535 w542] -> w512
          frame False {
            n197 = call "update action configuration.vi"("action config"=w541, "error in (no error)"=w537, "index"=w539, "sequence name"=w538, "Simple Sequencer TBM configuration in"=w540) -> ("error out"=w535:errorcluster, "Simple Sequencer TBM configuration out"=w536:refnum<class "Simple Sequencer TBM configuration.lvclass">)  [unwired: 5 in]
          }
          frame True {
          }
        }
        n198 = property on="Actions" class="LstBox (strict)"() -> ("Item Names"=w524:string[])  [unwired: 2 in, 2 out]
        n199 = Index Array(array=w524, index=w516) -> (element=w526:string)
        n200 = Empty String/Path?(string/path=w526) -> (empty?=w527:bool)
        n201 = Select(t=T9."Disabled and Grayed Out" ("Disabled"), s=w527, f=T9."Enabled" ("Disabled")) -> (s? t:f=w528:T9)
        n202 = property on="delete action" class="Bool"("DisabledEnum"=w528) -> ()  [unwired: 2 in, 2 out]
        n203 = case shown="False" w527 {
          tunnel: w516 -> [w558 _]
          tunnel: [w544 w567] -> w533
          tunnel: [w563 w568] -> w510
          tunnel: [w545 w566] -> w525
          tunnel: w513 -> [w562 w568]
          tunnel: w512 -> [w561 w567]
          tunnel: w526 -> [w546 _]
          tunnel: w520 -> [w548 w566]
          tunnel: w524 -> [w559 _]
          tunnel: [w551 T9."Disabled and Grayed Out" ("Disabled")] -> w522
          tunnel: [w550 T9."Disabled and Grayed Out" ("Disabled")] -> w523
          tunnel: w511 -> [w549 _]
          frame False {
            w553 = T9."Enabled" ("Disabled")
            w552 = T9."Disabled and Grayed Out" ("Disabled")
            n204 = Equal To 0?(x=w558) -> (x = 0?=w554:bool)
            n205 = Array Size(array=w559) -> (size(s)=w557:i32)
            n206 = call "get sequence action by index.vi"("error in (no error)"=w561, "index"=w558, "sequence name"=w549, "Simple Sequencer TBM configuration in"=w562) -> ("error out"=w560:errorcluster, "action configuration"=w547:refnum<class "action configuration.lvclass">, "Simple Sequencer TBM configuration out"=w563:refnum<class "Simple Sequencer TBM configuration.lvclass">)  [unwired: 5 in]
            n207 = Increment(x=w558) -> (x+1=w556:i32)
            n208 = Equal?(x=w556, y=w557) -> (x = y?=w555:bool)
            n209 = call "run action UI.vi"("error in (no error)"=w560, "action display name"=w546, "action configuration"=w547, "subpanel state"=w548) -> ("error out"=w544:errorcluster, "subpanel state out"=w545:T4)  [unwired: 6 in]
            n210 = Select(t=w552, s=w555, f=w553) -> (s? t:f=w550:T9)
            n211 = Select(t=w552, s=w554, f=w553) -> (s? t:f=w551:T9)
          }
          frame True {
          }
        }
        n212 = property on="Down Button" class="Bool"("DisabledEnum"=w523) -> ()  [unwired: 2 in, 2 out]
        n213 = property on="Up Button" class="Bool"("DisabledEnum"=w522) -> ()  [unwired: 2 in, 2 out]
      }
      event "Shutdown Action": Value Change {
        n214 = event-data() -> ()  [unwired: 1 in, 1 out]
        n215 = local read "Sequences"() -> (w585:i32)
        n216 = local read "Actions"() -> (w576:i32)
        n217 = property on="Sequences" class="LstBox (strict)"() -> ("Item Names"=w584:string[])  [unwired: 2 in, 2 out]
        n218 = Index Array(array=w584, index=w585) -> (element=w577:string)
        n219 = call "unload subpanel.vi"("error in (no error)"=w583, "subpanel state"=w582) -> ("error out"=w580:errorcluster, "empty?"=w581:bool, "action configuration out"=w579:refnum<class "action configuration.lvclass">, "subpanel state out"=w570:T4)  [unwired: 6 in]
        n220 = case shown="False" w581 {
          tunnel: [w592 w594] -> w575
          tunnel: [w591 w593] -> w574
          tunnel: w580 -> [w590 w593]
          tunnel: w579 -> [w586 _]
          tunnel: w578 -> [w589 w594]
          tunnel: w577 -> [w588 _]
          tunnel: w576 -> [w587 _]
          frame False {
            n221 = call "update action configuration.vi"("action config"=w586, "error in (no error)"=w590, "index"=w587, "sequence name"=w588, "Simple Sequencer TBM configuration in"=w589) -> ("error out"=w591:errorcluster, "Simple Sequencer TBM configuration out"=w592:refnum<class "Simple Sequencer TBM configuration.lvclass">)  [unwired: 5 in]
          }
          frame True {
          }
        }
        n222 = Unbundle By Name(w570) -> ("supported actions list"=w569:T6[])
        n223 = call "configure shutdown action UI.vi"("error in (no error)"=w574, "supported actions list"=w569, "user event"=w571, "Simple Sequencer TBM configuration"=w575) -> ("error out"=w572:errorcluster, "Simple Sequencer TBM configuration"=w573:refnum<class "Simple Sequencer TBM configuration.lvclass">)  [unwired: 6 in]
      }
    }
    n224 = case shown="Error" w52 {
      selector: w52 -> [w58 w64]
      tunnel: [w59 w65] -> w51
      tunnel: w41 -> [w59 w65]
      tunnel: [w58 w62] -> w50
      tunnel: w48 -> [w57 w61]
      tunnel: [w57 w61] -> w40
      tunnel: w43 -> [w56 w60]
      tunnel: [w56 w60] -> w42
      frame No Error {
      }
      frame Error {
        # "#CodeRecommended Any errors should be handled within the generating case or here. Current default is to clear everything"
        n225 = call <vilib>:"Simple Error Handler.vi"("error in (no error)"=w64) -> ("error out"=w63:errorcluster)  [unwired: 4 in, 4 out]
        n226 = call <vilib>:"Clear Errors.vi"("error in (no error)"=w63) -> ("error out"=w62:errorcluster)  [unwired: 5 in, 1 out]
      }
    }
  }
  n227 = Unregister For Events(event registration refnum=w38, error in=w37) -> (error out=w35:errorcluster)
  n228 = call <vilib>:"Simple Error Handler.vi"("error in (no error)"=w35) -> ()  [unwired: 4 in, 5 out]
